vi "StopAcquisitionResponseRoutedMessage_Name.vi"() -> (1 "message name":string="CmsAcquisition.StopAcquisitionResponse")   [LabVIEW 2017, in "CmsAcquisition.lvlib"]
uses:
  <vilib>/addons/InsightCM/Devices/Shared/Cms/CmsAcquisition/CmsAcquisition.lvlib
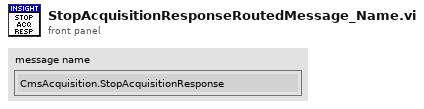
[diagram p1: front panel]
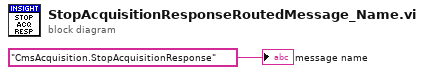
[diagram p0: block diagram]
diagram:
  "message name" <- "CmsAcquisition.StopAcquisitionResponse" ("ProcessName")
